vi "Slave VI.vi"() -> ()   [LabVIEW 2014]
panel:
  in  "stop":bool
  out "Vertical Progress Bar":u8(slide) scale=0.0..10.0
  out "led":bool
  # "SHARED VARIABLE"
  # "LED"
  # "PB"
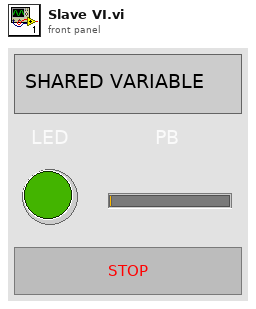
[diagram p1: front panel]
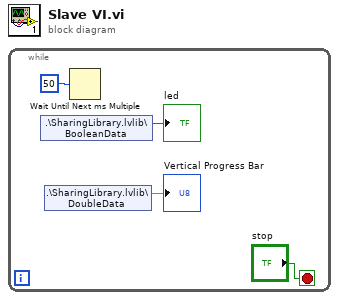
[diagram p0: block diagram]
diagram:
  n1 = while {
    stop <- "stop" stop-if-true
    n2 = shared-variable ".\\SharingLibrary.lvlib\\BooleanData"() -> (→"led":bool)  [unwired: 1 in, 1 out]
    n3 = shared-variable ".\\SharingLibrary.lvlib\\DoubleData"() -> (→"Vertical Progress Bar":dbl)  [unwired: 1 in, 1 out]
    n4 = Wait Until Next ms Multiple(millisecond multiple=u32 50) -> ()  [unwired: 1 out]
  }
